vi "RVC Quitic Polynomial Trajectory.vi"() -> ()   [LabVIEW 2013]
uses:
  <vilib>/Analysis/baseanly.llb/Mean (DBL).vi
  <vilib>/Analysis/NI_AALBase.lvlib
panel:
  out "mean by max":dbl
  out "velocity 2":cluster{dbl[], "P(A)":dbl[]}(graph)
  out "acceleration 2":cluster{dbl[], "P(A)":dbl[]}(graph)
  out "position 2":cluster{dbl[], "P(A)":dbl[]}(graph)
  out "velocity":cluster{dbl[], "P(A)":dbl[]}(graph)
  out "acceleration":cluster{dbl[], "P(A)":dbl[]}(graph)
  out "position":cluster{dbl[], "P(A)":dbl[]}(graph)
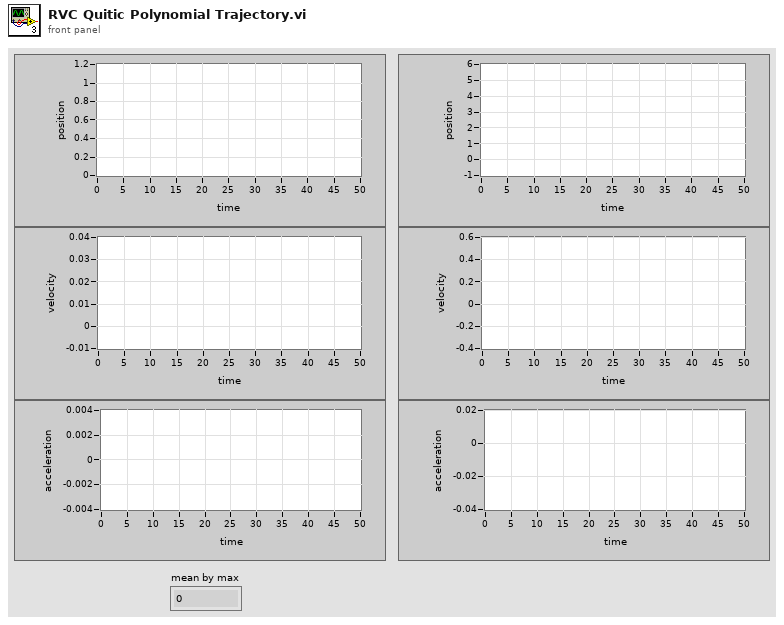
[diagram p1: front panel]
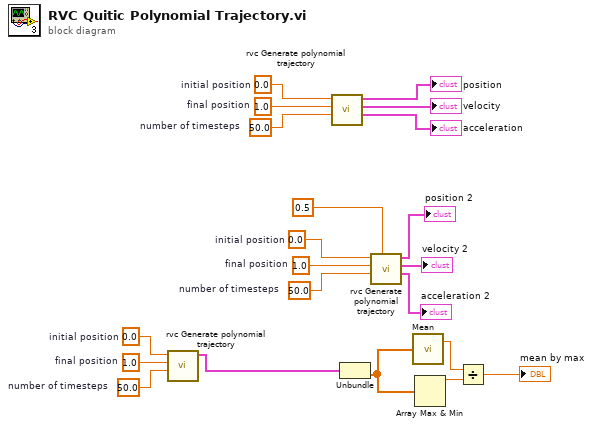
[diagram p0: block diagram]
diagram:
  w4 = 50.0  # number of timesteps
  w3 = 1.0  # final position
  w2 = 0.0  # initial position
  w16 = 50.0  # number of timesteps
  w15 = 1.0  # final position
  w14 = 0.0  # initial position
  w19 = 50.0  # number of timesteps
  w20 = 1.0  # final position
  w21 = 0.0  # initial position
  n1 = call "rvc Generate polynomial trajectory.vi"("number of timesteps"=w4, "final position"=w3, "initial position"=w2) -> ("position"=w1:cluster{dbl[], "P(A)":dbl[]})  [unwired: 6 in, 2 out]
  n2 = call "rvc Generate polynomial trajectory.vi"("number of timesteps"=w19, "final position"=w20, "initial position"=w21) -> ("acceleration"=→"acceleration":cluster{dbl[], "P(A)":dbl[]}, "velocity"=→"velocity":cluster{dbl[], "P(A)":dbl[]}, "position"=→"position":cluster{dbl[], "P(A)":dbl[]})  [unwired: 6 in]
  n3 = Unbundle(w1) -> ("P(A)"=w9:dbl[])  [unwired: 1 out]
  n4 = call "rvc Generate polynomial trajectory.vi"("initial velocity"=0.5, "number of timesteps"=w16, "final position"=w15, "initial position"=w14) -> ("acceleration"=→"acceleration 2":cluster{dbl[], "P(A)":dbl[]}, "velocity"=→"velocity 2":cluster{dbl[], "P(A)":dbl[]}, "position"=→"position 2":cluster{dbl[], "P(A)":dbl[]})  [unwired: 5 in]
  n5 = call-poly <vilib>:"Mean.vi"("X"=w9) -> ("mean"=w8:dbl)  [unwired: 1 out]
  n6 = Array Max & Min(array=w9) -> (max value=w7:dbl)  [unwired: 3 out]
  n7 = Divide(x=w8, y=w7) -> (x/y=→"mean by max":dbl)
